vi "dvp Vi Set Input Io Function.vi"(9 "InputIoFunction":u32(ring)=32769 items=["INPUT_FUNCTION_NORMAL"=32769, "INPUT_FUNCTION_TRIGGER"=32770], 10 "inputIo":u32(ring)=32769 items=["INPUT_IO_1"=32769, "INPUT_IO_2"=32770, "INPUT_IO_3"=32771, "INPUT_IO_4"=32772, "INPUT_IO_5"=32773, "INPUT_IO_6"=32774, "INPUT_IO_7"=32775, "INPUT_IO_8"=32776], 11 "handle":u32) -> (3 "function return":u32(ring))   [LabVIEW 2018, in "LabViewDVPCamera.lvlib"]
doc: "LabviewDvp2Api dvpStatus dvpViSetInputIoFunction(dvpHandle handle, dvpInputIo inputIo, dvpInputIoFunction InputIoFunction);"
uses:
  LabViewDVPCamera.lvlib
  LabViewDVPCamera/LabViewDVPCamera.dll
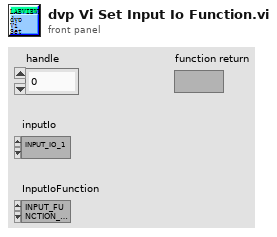
[diagram p1: front panel]
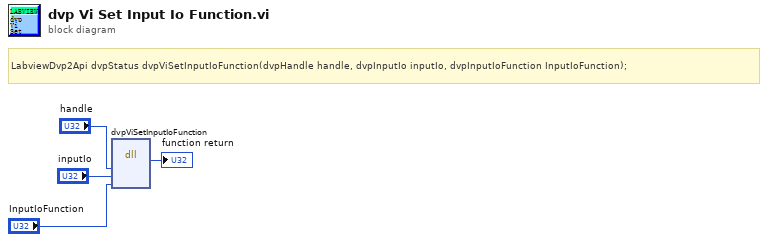
[diagram p0: block diagram]
diagram:
  # "LabviewDvp2Api dvpStatus dvpViSetInputIoFunction(dvpHandle handle, dvpInputIo inputIo, dvpInputIoFunction InputIoFunction);"
  n1 = dll-call lib="C:/Program Files (x86)/DVP2 Labview cn 64/Sample/LabViewDVPCamera/LabViewDVPCamera.*" fn="dvpViSetInputIoFunction"("handle"="handle", "inputIo"="inputIo", "InputIoFunction"="InputIoFunction") -> (→"function return":u32)  [unwired: 6 in, 2 out]
